vi "Get WIFI Name and Password.vi"(11 "WIFI Name":string) -> (0 "Target User WIFI Info":string, 1 "All WIFI Name Info":string, 2 "WIFI Name List":string[](array[string]), 3 "WIFI Password":string)   [LabVIEW 2015]
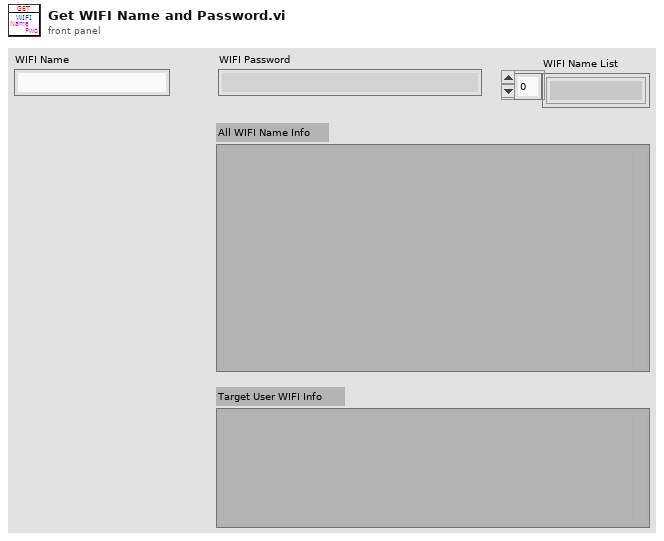
[diagram p1: front panel]
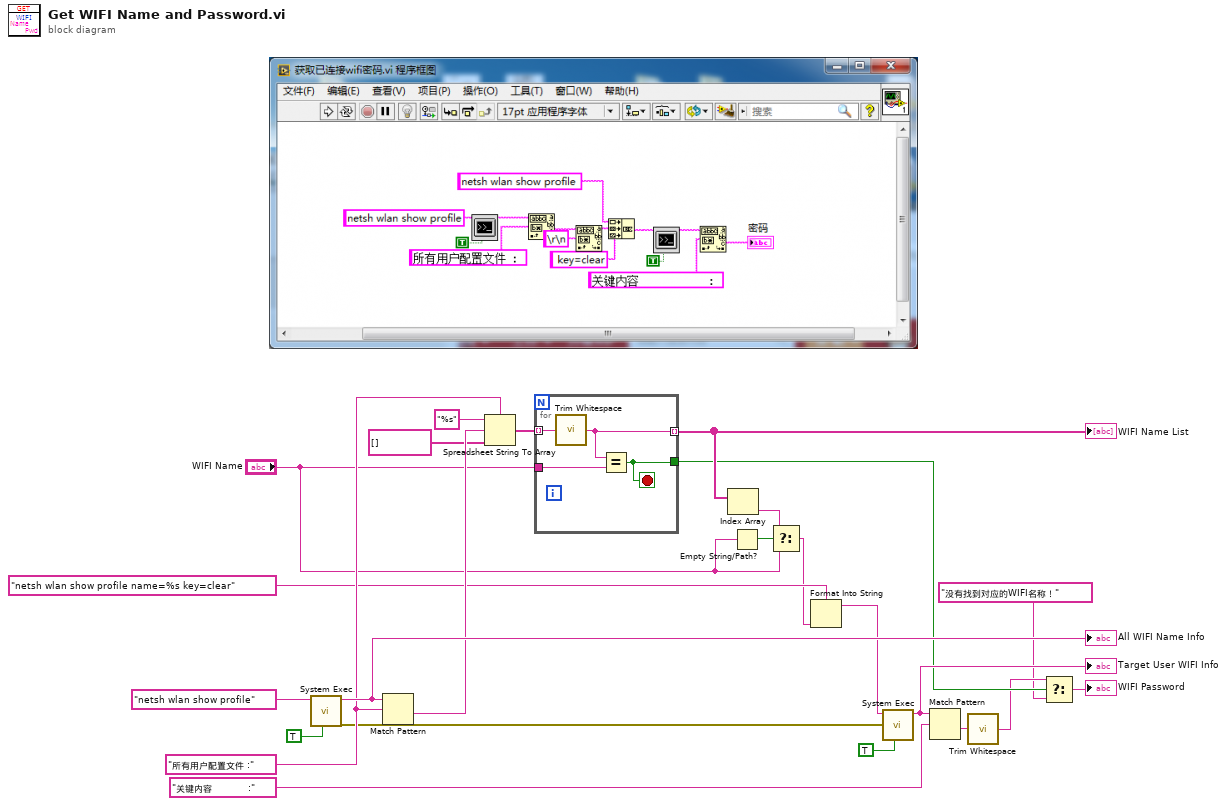
[diagram p0: block diagram]
diagram:
  w14 = "所有用户配置文件 :" ("regular expression")
  n1 = call <vilib>:"System Exec.vi"("run minimized? (F)"=TRUE, "command line"="netsh wlan show profile") -> ("error out"=w10:errorcluster, "standard output"=w22:string)  [unwired: 6 in, 2 out]
  "All WIFI Name Info" <- w22
  n2 = Match Pattern(string=w22, regular expression=w14) -> (after substring=w17:string)  [unwired: 1 in, 3 out]
  n3 = Spreadsheet String To Array(delimiter (Tab)=w14, format string="%s", spreadsheet string=w17, array type (2D Dbl)=string[] []) -> (array=w13:string[])
  n4 = for {
    tunnel: "WIFI Name" -> [w27]
    tunnel: w13 -> [w28] mode=indexing
    tunnel: [w26] -> w4
    tunnel: [w25] -> w7 mode=indexing
    stop <- w26 stop-if-true
    n5 = call <vilib>:"Trim Whitespace.vi"("string"=w28) -> ("trimmed string"=w25:string)  [unwired: 1 in]
    n6 = Equal?(x=w25, y=w27) -> (x = y?=w26:bool)
  }
  "WIFI Name List" <- w7
  n7 = Index Array(array=w7) -> (element=w8:string)  [unwired: 1 in]
  n8 = Empty String/Path?(string/path="WIFI Name") -> (empty?=w9:bool)
  n9 = Select(t=w8, s=w9, f="WIFI Name") -> (s? t:f=w6:string)
  n10 = Format Into String(format string="netsh wlan show profile name=%s key=clear" ("string"), w6) -> (resulting string=w11:string)  [unwired: 2 in, 1 out]
  n11 = call <vilib>:"System Exec.vi"("run minimized? (F)"=TRUE, "error in (no error)"=w10, "command line"=w11) -> ("standard output"=w20:string)  [unwired: 5 in, 3 out]
  "Target User WIFI Info" <- w20
  n12 = Match Pattern(string=w20, regular expression="关键内容            :") -> (after substring=w18:string)  [unwired: 1 in, 3 out]
  n13 = call <vilib>:"Trim Whitespace.vi"("string"=w18) -> ("trimmed string"=w3:string)  [unwired: 1 in]
  n14 = Select(t=w3, s=w4, f="没有找到对应的WIFI名称！" ("format string")) -> (s? t:f=→"WIFI Password":string)
